vi "DSF.Engine.Transfer Group.Get Direction.vi"(11 "Transfer Group in":refnum<class "DSF.Engine.Transfer Group.lvclass">) -> (2 "Direction":T1, 3 "Transfer Group out":refnum<class "DSF.Engine.Transfer Group.lvclass">)   [LabVIEW 2017, in "Data Sharing Framework Engine.lvlib" / "DSF.Engine.Transfer Group.lvclass"]
uses:
  DSF.Engine.Transfer Group.lvclass
  Source/Data Sharing Framework Core/Configuration/1.0.0/Public/Controls/DSF Direction.ctl
  DSF.Engine.Transfer Group.lvclass/DSF.Engine.Transfer Group.ctl
  Source/Data Sharing Framework Core/Configuration/1.0.0/Data Sharing Framework Configuration.lvlib
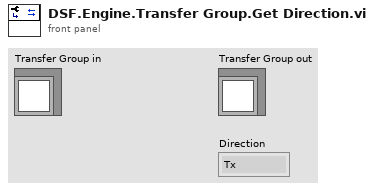
[diagram p1: front panel]
types:
  T1 = typedef "Data Sharing Framework Configuration.lvlib/DSF Direction.ctl" = enum8{"Tx", "Rx"}
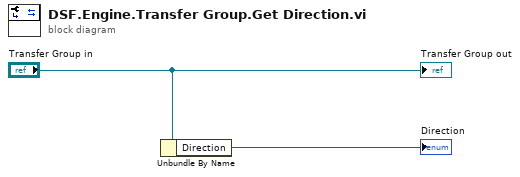
[diagram p0: block diagram]
diagram:
  n1 = Unbundle By Name("Transfer Group in") -> ("Direction"=→"Direction":T1)
  "Transfer Group out" <- "Transfer Group in"
